vi "数采仪日志报警存储(子VI).vi"   [LabVIEW 2016, in "数据传输系统-02.lvlib"]
types:
  T1 = cluster{"时间标识":timestamp, "设备":string, "日志信息":string, "流程参数":string}
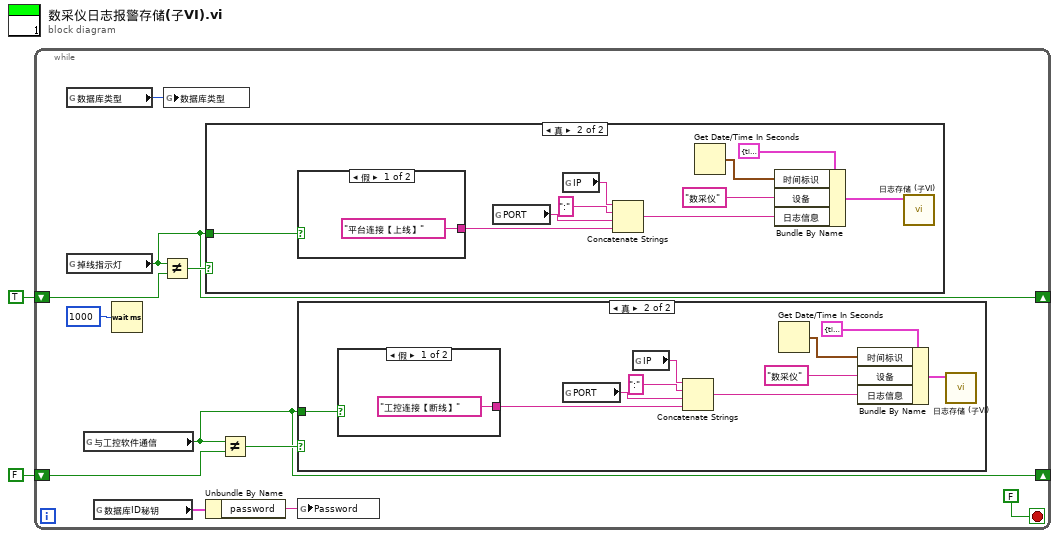
[diagram p0: block diagram]
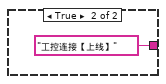
[diagram p3: hidden frame]
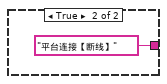
[diagram p5: hidden frame]
diagram:
  n1 = while {
    shift-right: [w9] -> _
    shift-left: TRUE -> [w10]
    shift-right: [w6] -> _
    shift-left: FALSE -> [w7]
    stop <- FALSE stop-if-true
    n2 = global read "断电保存全局.vi" "数据库类型"() -> (w3:enum16{"Access", "SQLite"})
    n3 = global read "全局 数据发送重叠.vi" "掉线指示灯"() -> (w9:bool)
    n4 = global read "全局1.vi" "与工控软件通信"() -> (w6:bool)
    n5 = global read "外部交互全局.vi" "数据库ID秘钥"() -> (w5:cluster{"userID":string, "password":string})
    n6 = Wait (ms)(milliseconds to wait=u32 1000 ("等待时间（毫秒）")) -> ()  [unwired: 1 out]
    n7 = Not Equal?(x=w9, y=w10) -> (x != y?=w11:bool)
    n8 = global write "外部调用接口全局变量.vi" "数据库类型"(w3) -> ()
    n9 = case shown="真" w11 {
      tunnel: w9 -> [_ w31]
      frame False {
      }
      frame True {
        n10 = case shown="假" w31 {
          tunnel: ["平台连接【上线】" ("设备") "平台连接【断线】" ("设备")] -> w27
          frame False {
          }
          frame True {
          }
        }
        n11 = global read "断电保存全局.vi" "PORT"() -> (w28:string)
        n12 = global read "断电保存全局.vi" "IP"() -> (w30:string)
        n13 = Concatenate Strings(w30, ":", w28, w27) -> (w26:string)
        n14 = Get Date/Time In Seconds() -> (seconds since 1Jan1904=w33:timestamp)
        n15 = Bundle By Name(cluster=T1 {"时间标识"=timestamp(0 s since 1904-01-01), "设备"="", "日志信息"="", "流程参数"=""} ("data in"), "时间标识"=w33, "设备"="数采仪", "日志信息"=w26) -> (w34:T1)
        n16 = call "日志存储 (子VI).vi"("data in"=w34) -> ()  [unwired: 11 in]
      }
    }
    n17 = Unbundle By Name(w5) -> ("password"=w4:string)
    n18 = Not Equal?(x=w6, y=w7) -> (x != y?=w8:bool)
    n19 = case shown="真" w8 {
      tunnel: w6 -> [_ w19]
      frame False {
      }
      frame True {
        n20 = case shown="假" w19 {
          tunnel: ["工控连接【断线】" ("设备") "工控连接【上线】" ("设备")] -> w14
          frame False {
          }
          frame True {
          }
        }
        n21 = global read "断电保存全局.vi" "PORT"() -> (w15:string)
        n22 = global read "断电保存全局.vi" "IP"() -> (w18:string)
        n23 = Concatenate Strings(w18, ":", w15, w14) -> (w17:string)
        n24 = Get Date/Time In Seconds() -> (seconds since 1Jan1904=w21:timestamp)
        n25 = Bundle By Name(cluster=T1 {"时间标识"=timestamp(0 s since 1904-01-01), "设备"="", "日志信息"="", "流程参数"=""} ("data in"), "时间标识"=w21, "设备"="数采仪", "日志信息"=w17) -> (w22:T1)
        n26 = call "日志存储 (子VI).vi"("data in"=w22) -> ()  [unwired: 11 in]
      }
    }
    n27 = global write "外部调用接口全局变量.vi" "Password"(w4) -> ()
  }
